vi "Read Config.vi"(8 "error in (no error)":errorcluster) -> (0 "error out":errorcluster, 3 "value":cluster{"Boolean text":string, "Value":i32}[](array[cluster]))   [LabVIEW 2020, in "Monedas.lvlib"]
doc: "Read configuration \n_____\nCreated using Delacor QMH Event Scripter 5.0.0.112."
uses:
  Monedas.lvlib
  <vilib>/Utility/xml.llb/Read From XML File(string).vi
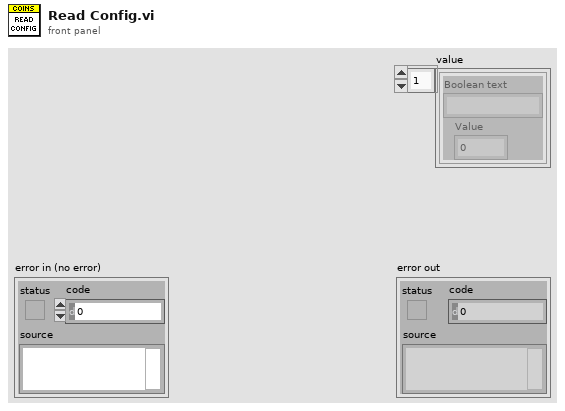
[diagram p1: front panel]
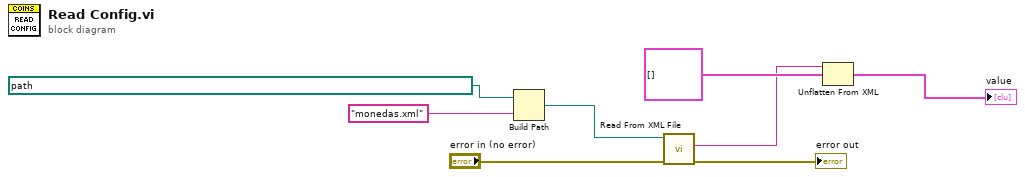
[diagram p0: block diagram]
diagram:
  n1 = Build Path(base path=path "C:/Users/Ymata/Desktop/séptimo/labview 7mo/Proyecto máuina/Proyecto-maquina", name or relative path="monedas.xml") -> (appended path=w7:path)
  n2 = call-poly <vilib>:"Read From XML File.vi"("error in (no error)"="error in (no error)", "XML File Path"=w7) -> ("error out"=→"error out":errorcluster, "XML Elements"=w1:string)  [unwired: 7 in, 1 out]
  n3 = Unflatten From XML(xml string=w1, type=cluster{"Boolean text":string, "Value":i32}[] []) -> (value=→"value":cluster{"Boolean text":string, "Value":i32}[])  [unwired: 1 in, 1 out]
